vi "Uncolour Info Table.vi"(8 "Error In":errorcluster, 11 "UI control refnums":T1) -> (0 "Error Out":errorcluster)   [LabVIEW 2012]
doc: "SciScan 1.2 160622\nThis VI restores the cell background colour of rows to grey.\nSince the number of rows calculated from no of tags in teh created macro, this VI must be called before carrying out a macro modification operation such as add/remove/reorder."
uses:
  Custom Controls and Typedefs/Macro_MD_UI Control Refnums.ctl
  Custom Controls and Typedefs/Delete Button.ctl
  Custom Controls and Typedefs/Edit Button.ctl
  Custom Controls and Typedefs/Timing Estimate Cluster.ctl
  CommonResource VIs/Timing/Timing Indicator.ctl
  Custom Controls and Typedefs/Load from PSM Button.ctl
  <vilib>/Utility/miscctls.llb/LVRowAndColumnTypeDef.ctl
panel:
  # "(hh:mm:ss)"
  # "(hh:mm:ss)"
  # "(hh:mm:ss)"
  # "(hh:mm:ss)"
  # "(hh:mm:ss)"
  # "(hh:mm:ss)"
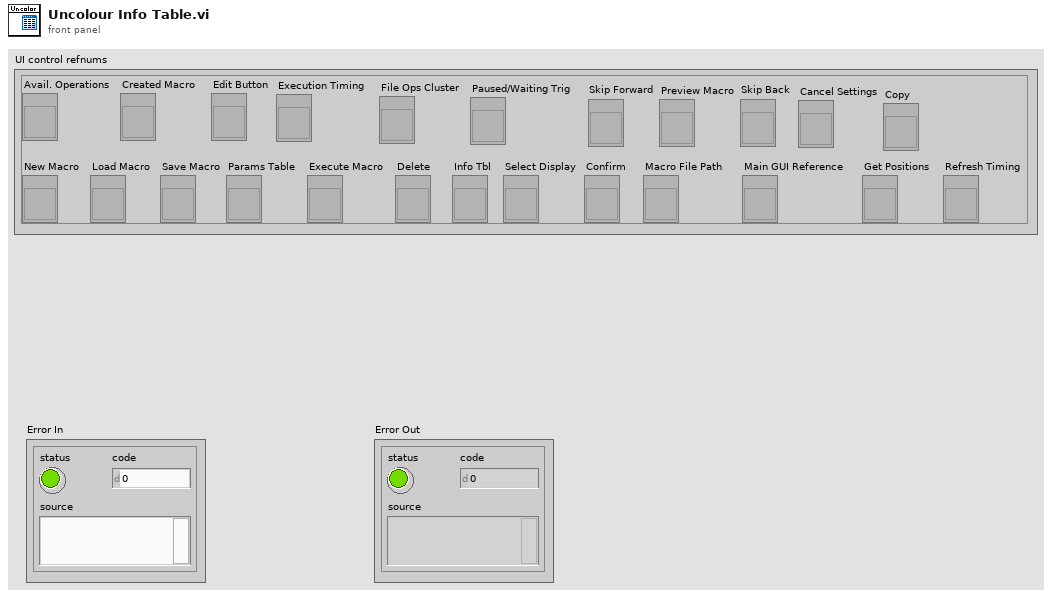
[diagram p1: front panel]
types:
  T1 = typedef "Macro_MD_UI Control Refnums.ctl" = cluster{"Avail. Operations":refnum<vi>, "Created Macro":refnum<vi>, "Load Macro":refnum<vi>, "Save Macro":refnum<vi>, "Params Table":refnum<vi>, "Delete":refnum<vi>, "Edit Button":refnum<vi>, "Execute Macro":refnum<vi>, "Info Tbl":refnum<vi>, "Execution Timing":refnum<vi>, "Select Display":refnum<vi>, "File Ops Cluster":refnum<vi>, "Paused/Waiting Trig":refnum<vi>, "Confirm":refnum<vi>, "New Macro":refnum<vi>, "Preview Macro":refnum<vi>, "Skip Forward":refnum<vi>, "Skip Back":refnum<vi>, "Macro File Path":refnum<vi>, "Main GUI Reference":refnum<vi>, "Cancel Settings":refnum<vi>, "Get Positions":refnum<vi>, "Copy":refnum<vi>, "Refresh Timing":refnum<vi>}
  T2 = typedef "LVRowAndColumnTypeDef.ctl" = cluster{"Row":i32, "Column":i32}
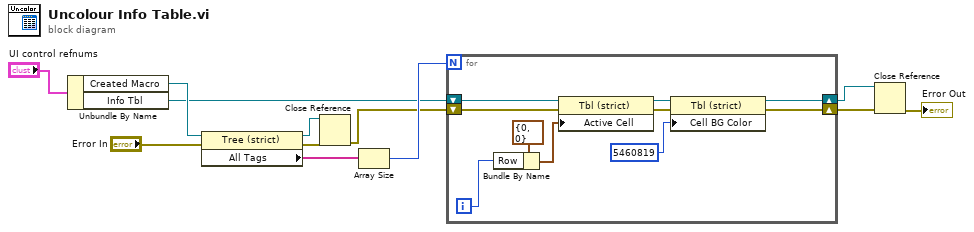
[diagram p0: block diagram]
diagram:
  n1 = Unbundle By Name("UI control refnums") -> ("Created Macro"=w11:refnum<vi>, "Info Tbl"=w6:refnum<vi>)
  n2 = property class="Tree (strict)"(reference=w11, error in="Error In") -> (reference out=w9:refnum<vi>, error out=w10:errorcluster, "All Tags"=w8:string[])
  n3 = Close Reference(reference=w9, error in (no error)=w10) -> (error out=w5:errorcluster)
  n4 = Array Size(array=w8) -> (size(s)=w7:i32)
  n5 = for {
    N: w7 -> [_]
    shift-right: [w14] -> w4
    shift-left: w6 -> [w17]
    shift-right: [w13] -> w3
    shift-left: w5 -> [w16]
    i -> [w15]
    n6 = Bundle By Name(cluster=T2 {"Row"=0, "Column"=0} ("Active Cell:Active Cell"), "Row"=w15) -> (w21:T2)
    n7 = property class="Tbl (strict)"(reference=w17, error in=w16, "Active Cell"=w21) -> (reference out=w20:refnum<vi>, error out=w19:errorcluster)
    n8 = property class="Tbl (strict)"(reference=w20, error in=w19, "Cell BG Color"=u32 5460819 ("Active Cell:Cell Background Color")) -> (reference out=w14:refnum<vi>, error out=w13:errorcluster)
  }
  n9 = Close Reference(reference=w4, error in (no error)=w3) -> (error out=→"Error Out":errorcluster)
